vi "Word_Save_Document.vi"(0 "Word._Document":refnum<k7>, 5 "password":string, 7 "path":string, 11 "error in (no error)":errorcluster) -> (15 "error out":errorcluster)   [LabVIEW 2010, in "NI_ReportGenerationToolkit.lvlib"]
uses:
  <vilib>/addons/_office/NI_ReportGenerationToolkit.lvlib
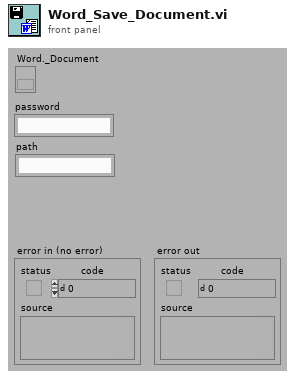
[diagram p1: front panel]
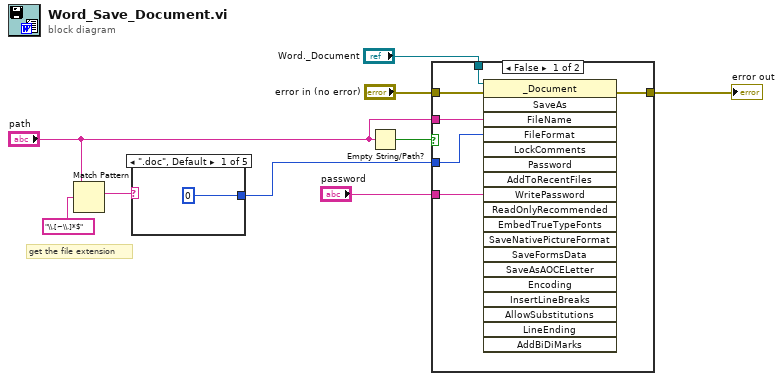
[diagram p0: block diagram]
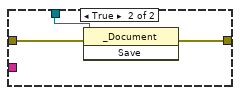
[diagram p2: hidden frame]
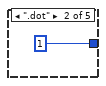
[diagram p3: hidden frame]
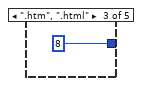
[diagram p4: hidden frame]
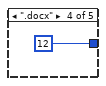
[diagram p5: hidden frame]
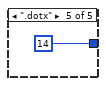
[diagram p6: hidden frame]
diagram:
  # "get the file extension"
  n1 = Match Pattern(string="path", regular expression="\\.[~\\.]*$") -> (match substring=w2:string)  [unwired: 4 out]
  n2 = case shown="\".doc\", Default" w2 {
    tunnel: [0 1 8 12 14] -> w1
    frame ".doc", Default {
    }
    frame ".dot" {
    }
    frame ".htm", ".html" {
    }
    frame ".docx" {
    }
    frame ".dotx" {
    }
  }
  n3 = Empty String/Path?(string/path="path") -> (empty?=w6:bool)
  n4 = case shown="False" w6 {
    tunnel: "Word._Document" -> [w20 w23]
    tunnel: "path" -> [w16 _]
    tunnel: "error in (no error)" -> [w19 w22]
    tunnel: [w18 w21] -> w9
    tunnel: "password" -> [w17 _]
    tunnel: w1 -> [w15 _]
    frame False {
      n5 = invoke class="_Document" method="SaveAs"(reference=w20, error in=w19, "FileName"=w16, "FileFormat"=w15, "WritePassword"=w17) -> (error out=w18:errorcluster)  [unwired: 14 in, 18 out]
    }
    frame True {
      n6 = invoke class="_Document" method="Save"(reference=w23, error in=w22) -> (error out=w21:errorcluster)  [unwired: 1 in, 2 out]
    }
  }
  "error out" <- w9
